vi "RSZVB Set Pulse Evaluation Mode.vi"(4 "Record Number (1)":i32=1, 5 "Evaluation Mode (0: Normal)":i32(ring) items=["Normal", "Mean"], 6 "Generator/Port Number (1)":i32=1, 7 "Interface Type (0: Generator)":i32(ring) items=["Generator", "Analyzer Source"], 8 "error in (no error)":errorcluster {"code" format="%.0x"}, 9 "Receiver Type (0: A)":i32(ring) items=["A", "B"], 10 "Channel (1)":i32=1, 11 "VISA session":refnum<visa-resource-name>) -> (0 "error out":errorcluster {"code" format="%.0x"}, 3 "dup VISA session":refnum<visa-resource-name>)   [LabVIEW 2011]
doc: "This VI specifies whether the wave quantity is displayed as measured or whether it is averaged. \n\nRemote-control command(s):\n[SENSe<Ch>:]PULSe:RECeiver:A<rec_no>:GENerator<gen_no>:EVALuation:MODE NORMal | MEAN\n[SENSe<Ch>:]PULSe:RECeiver:A<rec_no>:SRCPort<port_no>:EVALuation:MODE NORMal | MEAN\n[SENSe<Ch>:]PULSe:RECeiver:B<rec_no>:GENerator<gen_no>:EVALuation:MODE NORMal | MEAN\n[SENSe<Ch>:]PULSe:RECeiver:B<rec_no>:SRCPort<port_no>:EVALuation:MODE NORMal | MEAN"
uses:
  _utility/RSZVB Global Data.vi
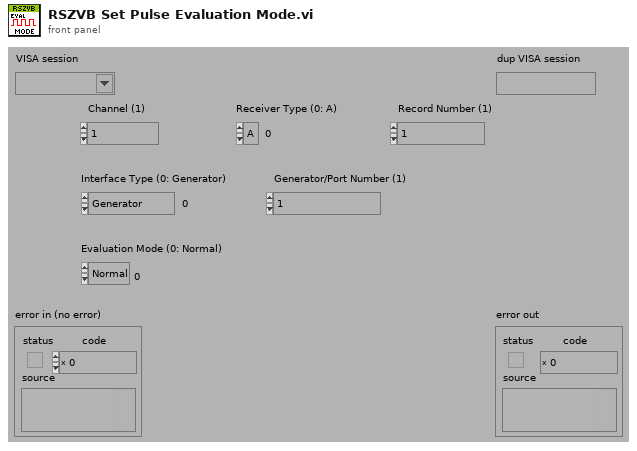
[diagram p1: front panel]
types:
  T1 = cluster{"Error Checking (T: On)":bool, "Installed Options":string[], "Data Valid?":bool, "Ports":i32, "Model":string[], "Option Checking (T: On)":bool}[]
  T2 = cluster{"Error Checking (T: On)":bool, "Installed Options":string[], "Data Valid?":bool, "Ports":i32, "Model":string[], "Option Checking (T: On)":bool}
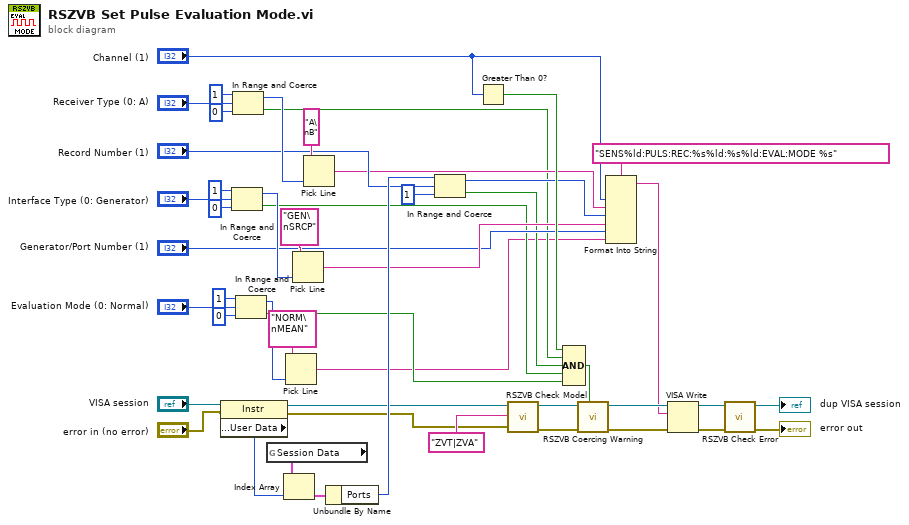
[diagram p0: block diagram]
diagram:
  n1 = property class="Instr"(reference="VISA session", error in="error in (no error)") -> (reference out=w16:refnum<visa-resource-name>, error out=w14:errorcluster, "General Settings:User Data"=w19:u32)
  n2 = In Range and Coerce(upper limit=1, x="Interface Type (0: Generator)", lower limit=0) -> (coerced(x)=w22:i32, In Range?=w5:bool)
  n3 = In Range and Coerce(upper limit=1, x="Receiver Type (0: A)", lower limit=0) -> (coerced(x)=w26:i32, In Range?=w7:bool)
  n4 = In Range and Coerce(upper limit=1, x="Evaluation Mode (0: Normal)", lower limit=0) -> (coerced(x)=w37:i32, In Range?=w4:bool)
  n5 = global read "RSZVB Global Data.vi" "Session Data"() -> (w20:T1)
  n6 = Index Array(array=w20, index=w19) -> (element=w21:T2)
  n7 = Pick Line(multi-line string="NORM\nMEAN", line index=w37) -> (output string=w1:string)  [unwired: 1 in]
  n8 = Pick Line(multi-line string="GEN\nSRCP", line index=w22) -> (output string=w9:string)  [unwired: 1 in]
  n9 = Pick Line(multi-line string="A\nB", line index=w26) -> (output string=w11:string)  [unwired: 1 in]
  n10 = Unbundle By Name(w21) -> ("Ports"=w18:i32)
  n11 = In Range and Coerce(upper limit=w18, x="Record Number (1)", lower limit=1) -> (coerced(x)=w10:i32, In Range?=w6:bool)
  n12 = Greater Than 0?(x="Channel (1)") -> (x > 0?=w41:bool)
  n13 = call "RSZVB Check Model.vi"("error in (no error)"=w14, "Model"="ZVT|ZVA" ("Options"), "VISA session"=w16) -> ("error out"=w33:errorcluster, "dup VISA session"=w32:refnum<visa-resource-name>)  [unwired: 7 in]
  n14 = Compound Arithmetic op=AND(w41, w7, w6, w5, w4) -> (w43:bool)
  n15 = call "RSZVB Coercing Warning.vi"("In Range?"=w43, "error in (no error)"=w33, "VISA session"=w32) -> ("error out"=w46:errorcluster, "dup VISA session"=w47:refnum<visa-resource-name>)  [unwired: 7 in]
  n16 = Format Into String(format string="SENS%ld:PULS:REC:%s%ld:%s%ld:EVAL:MODE %s", "Channel (1)", w11, w10, w9, "Generator/Port Number (1)", w1) -> (resulting string=w42:string)  [unwired: 2 in, 1 out]
  n17 = VISA Write(VISA resource name=w47, write buffer=w42, error in (no error)=w46) -> (VISA resource name out=w44:refnum<visa-resource-name>, error out=w45:errorcluster)  [unwired: 1 out]
  n18 = call "RSZVB Check Error.vi"("error in (no error)"=w45, "VISA session"=w44) -> ("error out"=→"error out":errorcluster, "dup VISA session"=→"dup VISA session":refnum<visa-resource-name>)  [unwired: 8 in]
